vi "CreateFileHandler.vi"(4 "Delay":bool, 6 "Errors":string, 7 "FIlePath":path, 8 "error in (no error)":errorcluster, 9 "Encoding":string, 10 "Mode":string, 11 "Logger in":refnum<class "Logger.lvclass">) -> (0 "error out":errorcluster, 2 "FileHandler":refnum<class "FileHandler.lvclass">, 3 "Logger out":refnum<class "Logger.lvclass">)   [LabVIEW 2022 SP3, in "Logger.lvlib" / "Logger.lvclass"]
uses:
  Logger.lvclass
  C:/Users/jakub/repos/gh/PythonWrapper/Source/PythonWrapper/PythonWrapper.lvclass
  PythonWrapper/Source/PythonWrapper/PythonWrapper.lvclass/PythonWrapper.ctl
  Logger.lvclass/Logger.ctl
  Handler/Handler.lvclass/Handler.ctl
  PythonWrapper/Source/PythonWrapper/Read PythonSession.vi
  PythonWrapper/Source/PythonWrapper/Read ModulePath.vi
  Read Logger.vi
  Handler/Write Name.vi
  Handler/Write Handler.vi
  FileHandler/FileHandler.lvclass
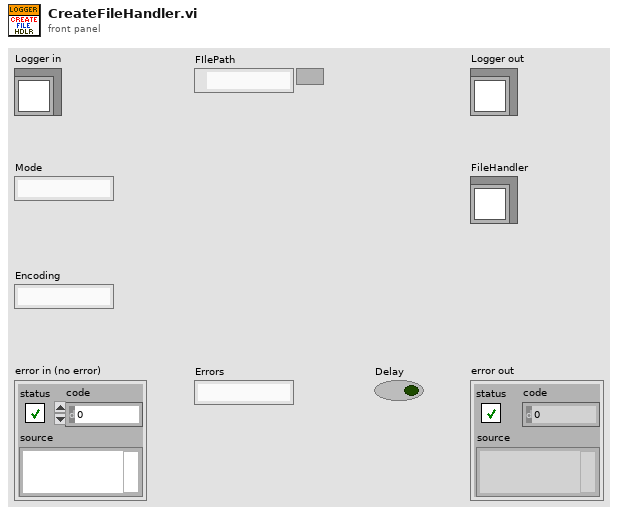
[diagram p1: front panel]
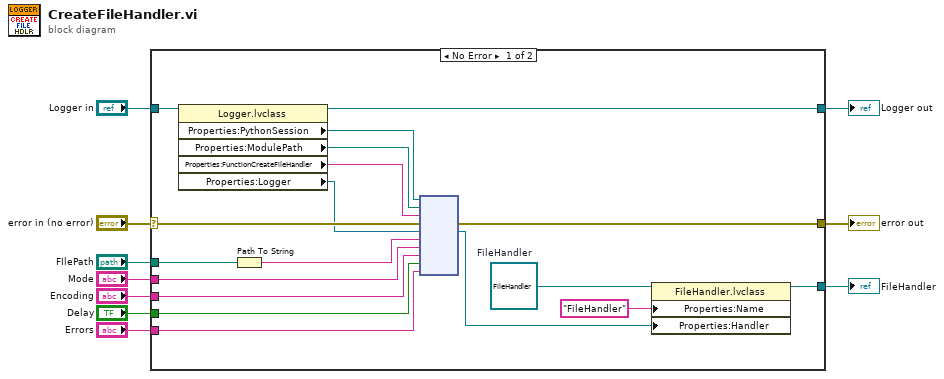
[diagram p0: block diagram]
diagram:
  n1 = case shown="No Error" "error in (no error)" {
    selector: "error in (no error)" -> [w26 w30]
    tunnel: [w15 w30] -> w7
    tunnel: [w27 w29] -> w9
    tunnel: "Logger in" -> [w28 w29]
    tunnel: "FIlePath" -> [w21 _]
    tunnel: "Mode" -> [w19 _]
    tunnel: "Encoding" -> [w18 _]
    tunnel: "Delay" -> [w17 _]
    tunnel: "Errors" -> [w16 _]
    tunnel: [w11 _] -> w1
    frame No Error {
      w14 = refnum<class "FileHandler.lvclass"> refnum  # FileHandler
      n2 = property class="Logger.lvclass"(reference=w28) -> (reference out=w27:refnum<class "Logger.lvclass">, "Properties:PythonSession"=w25:refnum<k35>, "Properties:ModulePath"=w23:path, "Properties:FunctionCreateFileHandler"=w24:string, "Properties:Logger"=w22:refnum<k38>)  [unwired: 1 in, 1 out]
      n3 = Path To String(path=w21) -> (string=w20:string)
      n4 = node(w25, w23, w24, w26, w22, w20, w19, w18, w17, w16) -> (w15:errorcluster, w12:refnum<k38>)  [unwired: 5 in, 3 out]
      n5 = property class="FileHandler.lvclass"(reference=w14, "Properties:Name"="FileHandler" ("Name"), "Properties:Handler"=w12) -> (reference out=w11:refnum<class "FileHandler.lvclass">)  [unwired: 1 in, 1 out]
    }
    frame Error {
    }
  }
  "error out" <- w7
  "Logger out" <- w9
  "FileHandler" <- w1
